vi "Close.vi"(8 "error in (no error)":errorcluster, 11 "Cluster of class private data":T1) -> (0 "error out":errorcluster)   [LabVIEW 2011]
uses:
  UDP Base.ctl
  UDP Socket Params.ctl
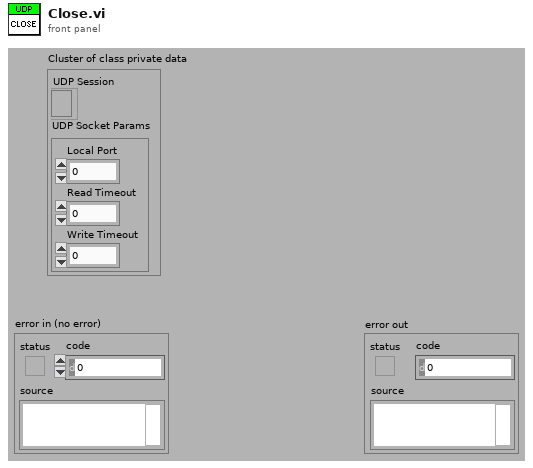
[diagram p1: front panel]
types:
  T1 = typedef "UDP Base.ctl" = cluster{"UDP Session":refnum<k16>, "UDP Socket Params":T2}
  T2 = typedef "UDP Socket Params.ctl" = cluster{"Local Port":u16, "Read Timeout":i32, "Write Timeout":i32}
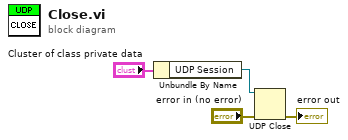
[diagram p0: block diagram]
diagram:
  n1 = Unbundle By Name("Cluster of class private data") -> ("UDP Session"=w4:refnum<k16>)
  n2 = UDP Close(connection ID=w4, 8:"error in (no error)") -> (error out=→"error out":errorcluster)  [unwired: 1 out]
